vi "ROI entry-Get image size.vi"(8 "error in (no error)":errorcluster) -> (0 "error out":errorcluster, 3 "Image size":cluster{"X Resolution":i32, "Y Resolution":i32})   [LabVIEW 2020]
uses:
  <vilib>/vision/Image Controls.llb/IMAQ Image.ctl
  Globals/gl_ROI Entry UI globals.vi
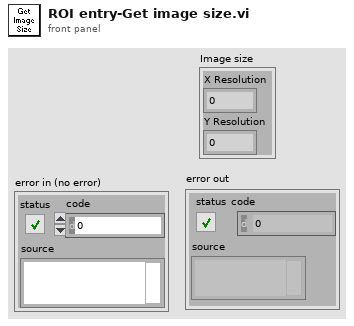
[diagram p1: front panel]
types:
  T1 = typedef "IMAQ Image.ctl" = refnum<image>
  T2 = typedef "ROI entry screen ctrl refs cluster.ctl" = cluster{"Done button":refnum<vi>, "Imaging button":refnum<vi>, "Acquisition button":refnum<vi>, "Scan dwell time per pixel (us)":refnum<vi>, "# of planes":refnum<vi>, "Zoom Ctrl":refnum<vi>, "Equal size":refnum<vi>, "Channel":refnum<vi>, "Image Display":refnum<vi>, "Z-Plane Selector":refnum<vi>, "Number of lines left":refnum<vi>, "Z-stack folder path":refnum<vi>, "POI Density":refnum<vi>, "Arb Plane Entry":refnum<vi>, "Whole Plane":refnum<vi>, "Line Mode":refnum<vi>, "Clear Last":refnum<vi>, "Clear All":refnum<vi>, "Delete Lines":refnum<vi>, "Trial Length (sec)":refnum<vi>, "Palette Type":refnum<vi>, "Intensity slider":refnum<vi>, "# POI":refnum<vi>, "Max Z Proj":refnum<vi>, "Zplane ind":refnum<vi>, "Wavelength (nm)":refnum<vi>, "Number of Trials":refnum<vi>, "Funct stim.trig.enable":refnum<vi>, "Funct stim.trig.delay (s)":refnum<vi>, "Line Mode":refnum<vi>, "Step size (µm)":refnum<vi>, "ROI move mode":refnum<vi>, "Cool-down time (s)":refnum<vi>, "Enable cool-down time":refnum<vi>, "Motor Z ind. (um)":refnum<vi>, "AOL Z ind. (um)":refnum<vi>, "Load Reference Image":refnum<vi>, "Rel.  Res.":refnum<vi>, "ROI LIST":refnum<vi>, "Show All":refnum<vi>, "ROI Type":refnum<vi>, "Start Plane":refnum<vi>, "Stop Plane":refnum<vi>, "Offset ROI":refnum<vi>, "Tab Control":refnum<vi>, "Laser Power(%)":refnum<vi>, "Cycle rate":refnum<vi>, "FOV (Ind.)":refnum<vi>, "Frame Size (Ind.)":refnum<vi>, "Resolution (Ind.)":refnum<vi>, "Pixel Density (Ind)":refnum<vi>, "Laser Power (Ind.)":refnum<vi>, "Dwell Time (Ind.)":refnum<vi>, "Adj MC":refnum<vi>}
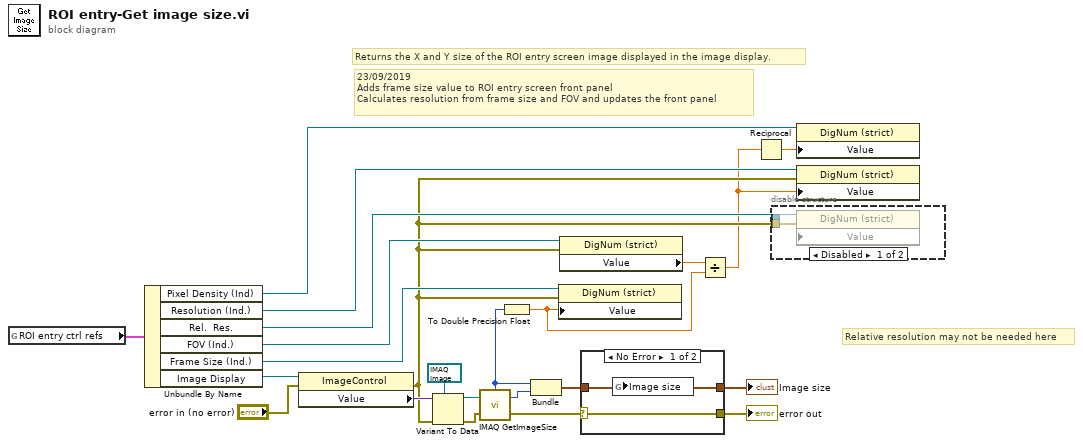
[diagram p0: block diagram]
diagram:
  # "Relative resolution may not be needed here"
  # "23/09/2019\nAdds frame size value to ROI entry screen front panel\nCalculates resolution from frame size and FOV and updates the front panel"
  # "Returns the X and Y size of the ROI entry screen image displayed in the image display."
  n1 = global read "gl_ROI Entry UI globals.vi" "ROI entry ctrl refs"() -> (w21:T2)
  n2 = Unbundle By Name(w21) -> ("Pixel Density (Ind)"=w3:refnum<vi>, "Resolution (Ind.)"=w5:refnum<vi>, "Rel.  Res."=w8:refnum<vi>, "FOV (Ind.)"=w9:refnum<vi>, "Frame Size (Ind.)"=w11:refnum<vi>, "Image Display"=w20:refnum<vi>)
  n3 = property on="Property Node" class="ImageControl"(reference=w20, error in="error in (no error)") -> (error out=w4:errorcluster, "Value"=w19:variant)  [unwired: 1 out]
  n4 = Variant To Data(error in=w4, type=T1 refnum ("element"), Variant=w19) -> (data=w17:T1, error out=w23:errorcluster)
  n5 = call "IMAQ GetImageSize"("Image"=w17, "error in (no error)"=w23) -> ("Y Resolution"=w22:i32, "X Resolution"=w10:i32, "error out"=w14:errorcluster)  [unwired: 2 in]
  n6 = To Double Precision Float(number=w10) -> (double precision float=w6:dbl)
  n7 = Bundle("X Resolution"=w10, "Y Resolution"=w22) -> (w16:cluster{"X Resolution":i32, "Y Resolution":i32})  [unwired: 1 in]
  n8 = property on="Property Node" class="DigNum (strict)"(reference=w11, error in=w4, "Value"=w6) -> ()  [unwired: 2 out]
  n9 = property on="Property Node" class="DigNum (strict)"(reference=w9, error in=w4) -> ("Value"=w7:dbl)  [unwired: 2 out]
  n10 = case shown="No Error" w14 {
    selector: w14 -> [w25 w27]
    tunnel: w16 -> [w24 w26]
    tunnel: [w25 w27] -> w13
    tunnel: [w24 w26] -> w12
    frame No Error {
      n11 = global write "gl_ROI Entry UI globals.vi" "Image size"(w24) -> ()
    }
    frame Error {
    }
  }
  "Image size" <- w12
  "error out" <- w13
  n12 = Divide(x=w7, y=w6) -> (x/y=w1:dbl)
  n13 = Reciprocal(x=w1) -> (1/x=w2:dbl)
  n14 = disable-structure shown="Disabled" {
    disable-tunnel: w8 -> [w29 _]
    disable-tunnel: w4 -> [w28 _]
    frame Disabled {
      n15 = property on="Property Node" class="DigNum (strict)" props=["Value"](reference=w29, error in=w28) -> ()  [unwired: 1 in, 2 out]
    }
    frame Enabled {
    }
  }
  n16 = property on="Property Node" class="DigNum (strict)"(reference=w3, "Value"=w2) -> ()  [unwired: 1 in, 2 out]
  n17 = property on="Property Node" class="DigNum (strict)"(reference=w5, error in=w4, "Value"=w1) -> ()  [unwired: 2 out]
